vi "correction_beamshaper_example.vi"() -> ()   [LabVIEW 2020, in "ILAO_BeamShaper.lvclass"]
uses:
  ILAO_BeamShaper/ILAO_BeamShaper.lvclass
  HASO4_3/WaveKit/Controls/InteractionMatrixToCommandMatrixParameters.ctl
  HASO4_3/WaveKit/Classes/CorrectionDataManager/CorrectionDataManager.lvclass
  HASO4_3/WaveKit/Classes/Pupil/Pupil.lvclass
  HASO4_3/WaveKit/Controls/Point2Df.ctl
  HASO4_3/WaveKit/Controls/CircularPupilDetectionParams.ctl
  HASO4_3/WaveKit/Controls/PupilDetectionOption.ctl
  HASO4_3/WaveKit/Controls/CircularAutoDetectionOptions.ctl
  HASO4_3/WaveKit/Controls/PupilDetectionMode.ctl
  HASO4_3/WaveKit/Controls/WavefrontModalReconstructionType.ctl
  HASO4_3/WaveKit/Classes/ModalCoef/ModalCoef.lvclass
  HASO4_3/WaveKit/Classes/ComputePhaseSet/ComputePhaseSet.lvclass
  HASO4_3/WaveKit/Controls/WavefrontReconstructionMode.ctl
  HASO4_3/WaveKit/Classes/HasoSlopes/HasoSlopes.lvclass
  HASO4_3/WaveKit/Classes/WavefrontCorrector/WavefrontCorrector.lvclass
  HASO4_3/WaveKit/Controls/ZernikeModalPrefs.ctl
  HASO4_3/WaveKit/Controls/ZernikeProjectionPupilSetup.ctl
panel:
  in  "Interaction matrix path 2":path
  in  "Haso config file path 2":path
  in  "PathToWavefrontCorrectorSetupFile 2":path
  out "Delta commands 2":sgl[](graph)
  in  "Prefs 2":T1={"Number of kept modes"=32, "Tilt filtering"=FALSE}
  in  "Zernike Value 2":dbl[](array[numeric])=[0.0, 0.0, 0.0, 0.0, 0.0, 0.0, 0.0, 0.0, 0.0]
  in  "Normalization 2":bool
  in  "set_init_state_from_config_file":bool
  in  "PathToWavefrontCorrectorSetupFile":path
  out "error out":errorcluster
  out "Delta commands":sgl[](graph)
  in  "Prefs":T1={"Number of kept modes"=32, "Tilt filtering"=FALSE}
  in  "Zernike Value":dbl[](array[numeric])=[0.0, 0.0, 0.0, 0.0, 0.0, 0.0, 0.0, 0.0, 0.0]
  in  "Normalization":bool
  in  "Interaction matrix path":path
  in  "Haso config file path":path
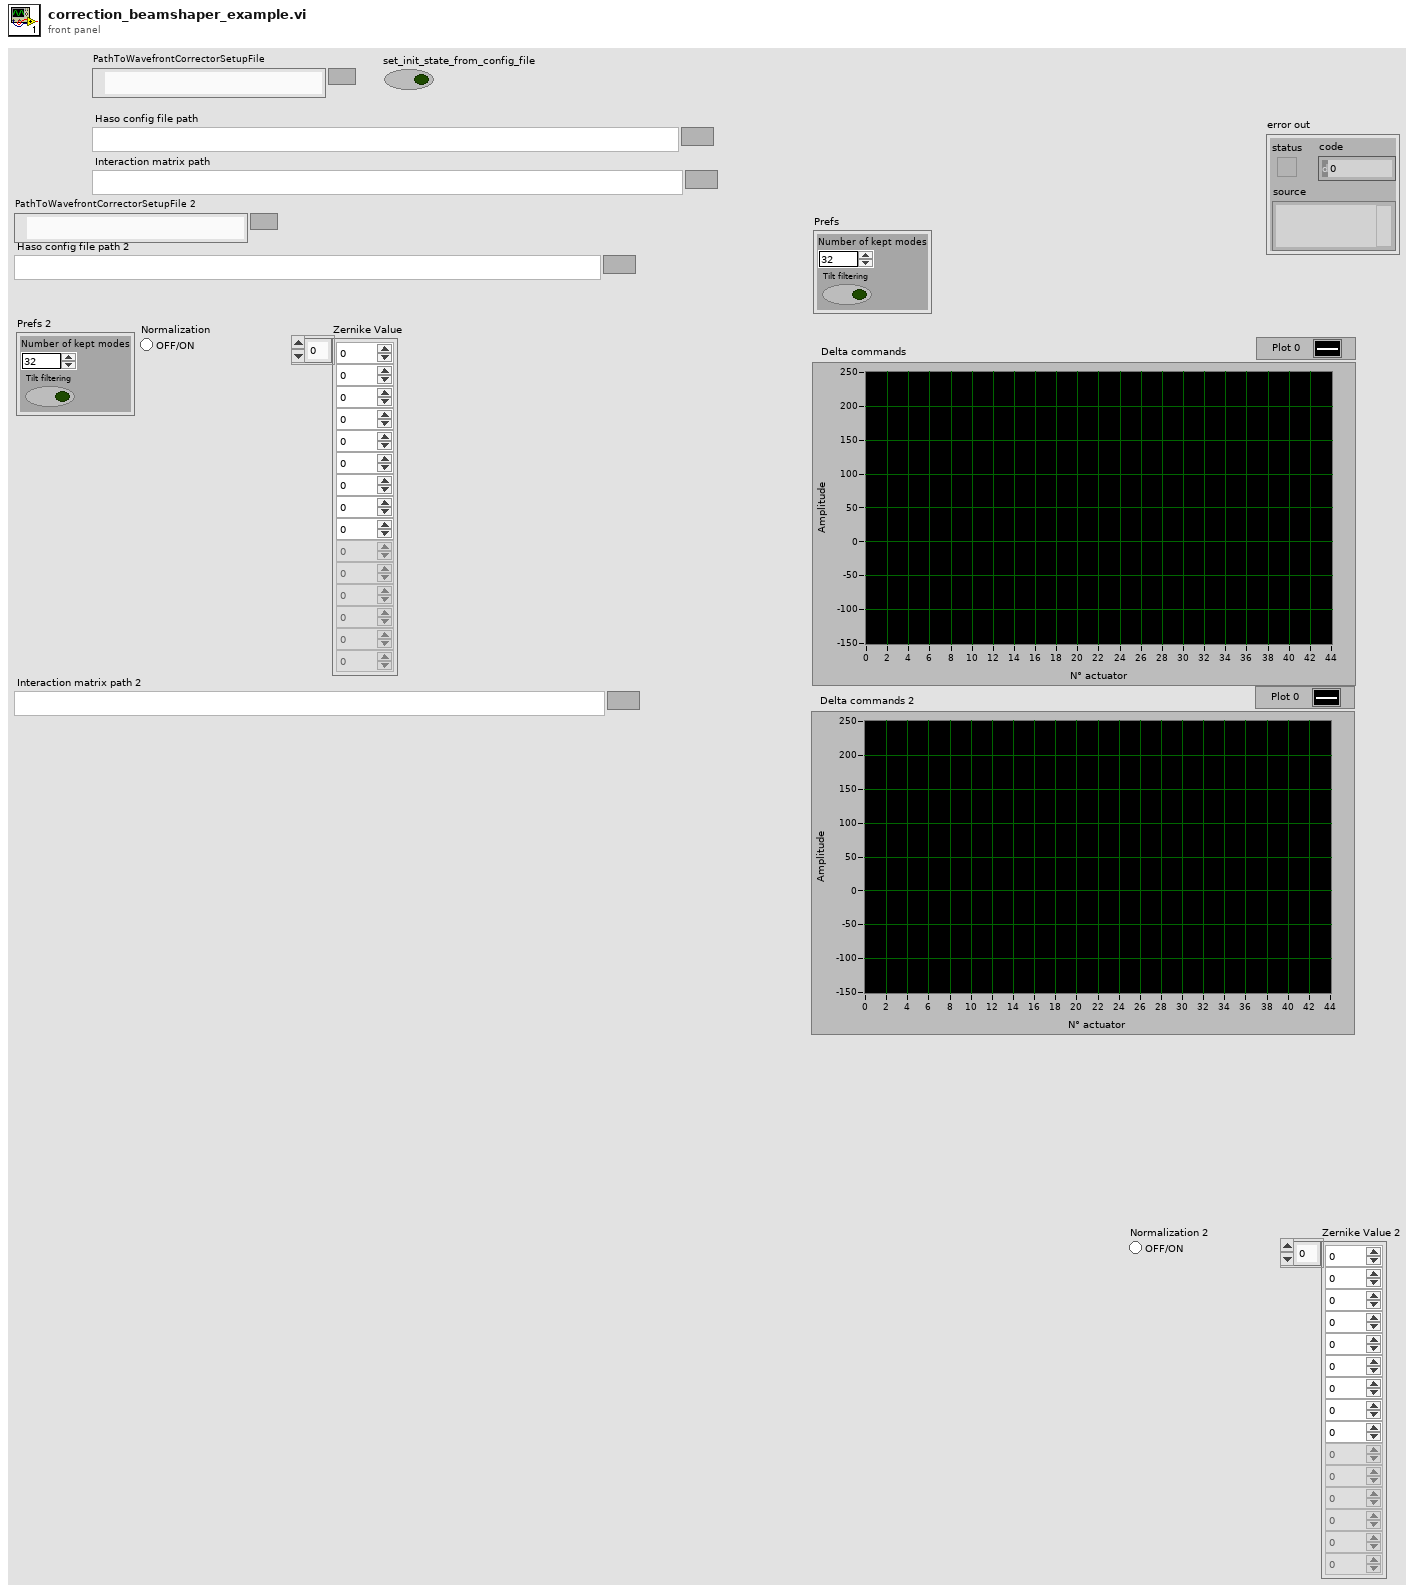
[diagram p1: front panel]
types:
  T1 = typedef "InteractionMatrixToCommandMatrixParameters.ctl" = cluster{"Number of kept modes":i32, "Tilt filtering":bool}
  T2 = typedef "ZernikeModalPrefs.ctl" = cluster{"Number of coefficients":u32, "Filtered coefficients":u32[], "RMS Zernike normalization":bool, "CircularProjectionPupilDimensions":T3}
  T3 = typedef "ZernikeProjectionPupilSetup.ctl" = cluster{"Pupil center_sspp":T4, "Pupil radius_sspp":sgl}
  T4 = typedef "Point2Df.ctl" = cluster{"X":sgl, "Y":sgl}
  T5 = typedef "WavefrontReconstructionMode.ctl" = enum16{"None", "Modal_Legendre", "Modal_Zernike", "Zonal", "Modal_Zonal_Zernike", "Modal_Zonal_Legendre"}
  T6 = typedef "WavefrontModalReconstructionType.ctl" = enum16{"Legendre", "Zernike"}
  T7 = typedef "CircularPupilDetectionParams.ctl" = cluster{"PupilDetectionOption":T8, "AutoDetectionOption":T9, "PupilDetectionMode":T10, "CentralOccultationDetection":bool}
  T8 = typedef "PupilDetectionOption.ctl" = enum16{"Manual", "Automatic"}
  T9 = typedef "CircularAutoDetectionOptions.ctl" = enum16{"manual_radius_auto_center", "manual_center_auto_radius", "auto_radius_auto_center"}
  T10 = typedef "PupilDetectionMode.ctl" = enum16{"inscribed", "circumscribed"}
  T11 = typedef "CasaoManagerGeneralSpecifications.ctl" = cluster{"Wavefront corrector name":string, "Wavefront corrector serial number":string, "Nb actuators":i32, "HASO serial number":string, "Dimension_um":T12}
  T12 = typedef "General dimensions definition.ctl" = cluster{"Size":T13, "Step":T4}
  T13 = typedef "Point2D.ctl" = cluster{"X":u32, "Y":u32}
  T14 = typedef "Wavefront Corrector Position.ctl" = sgl[]
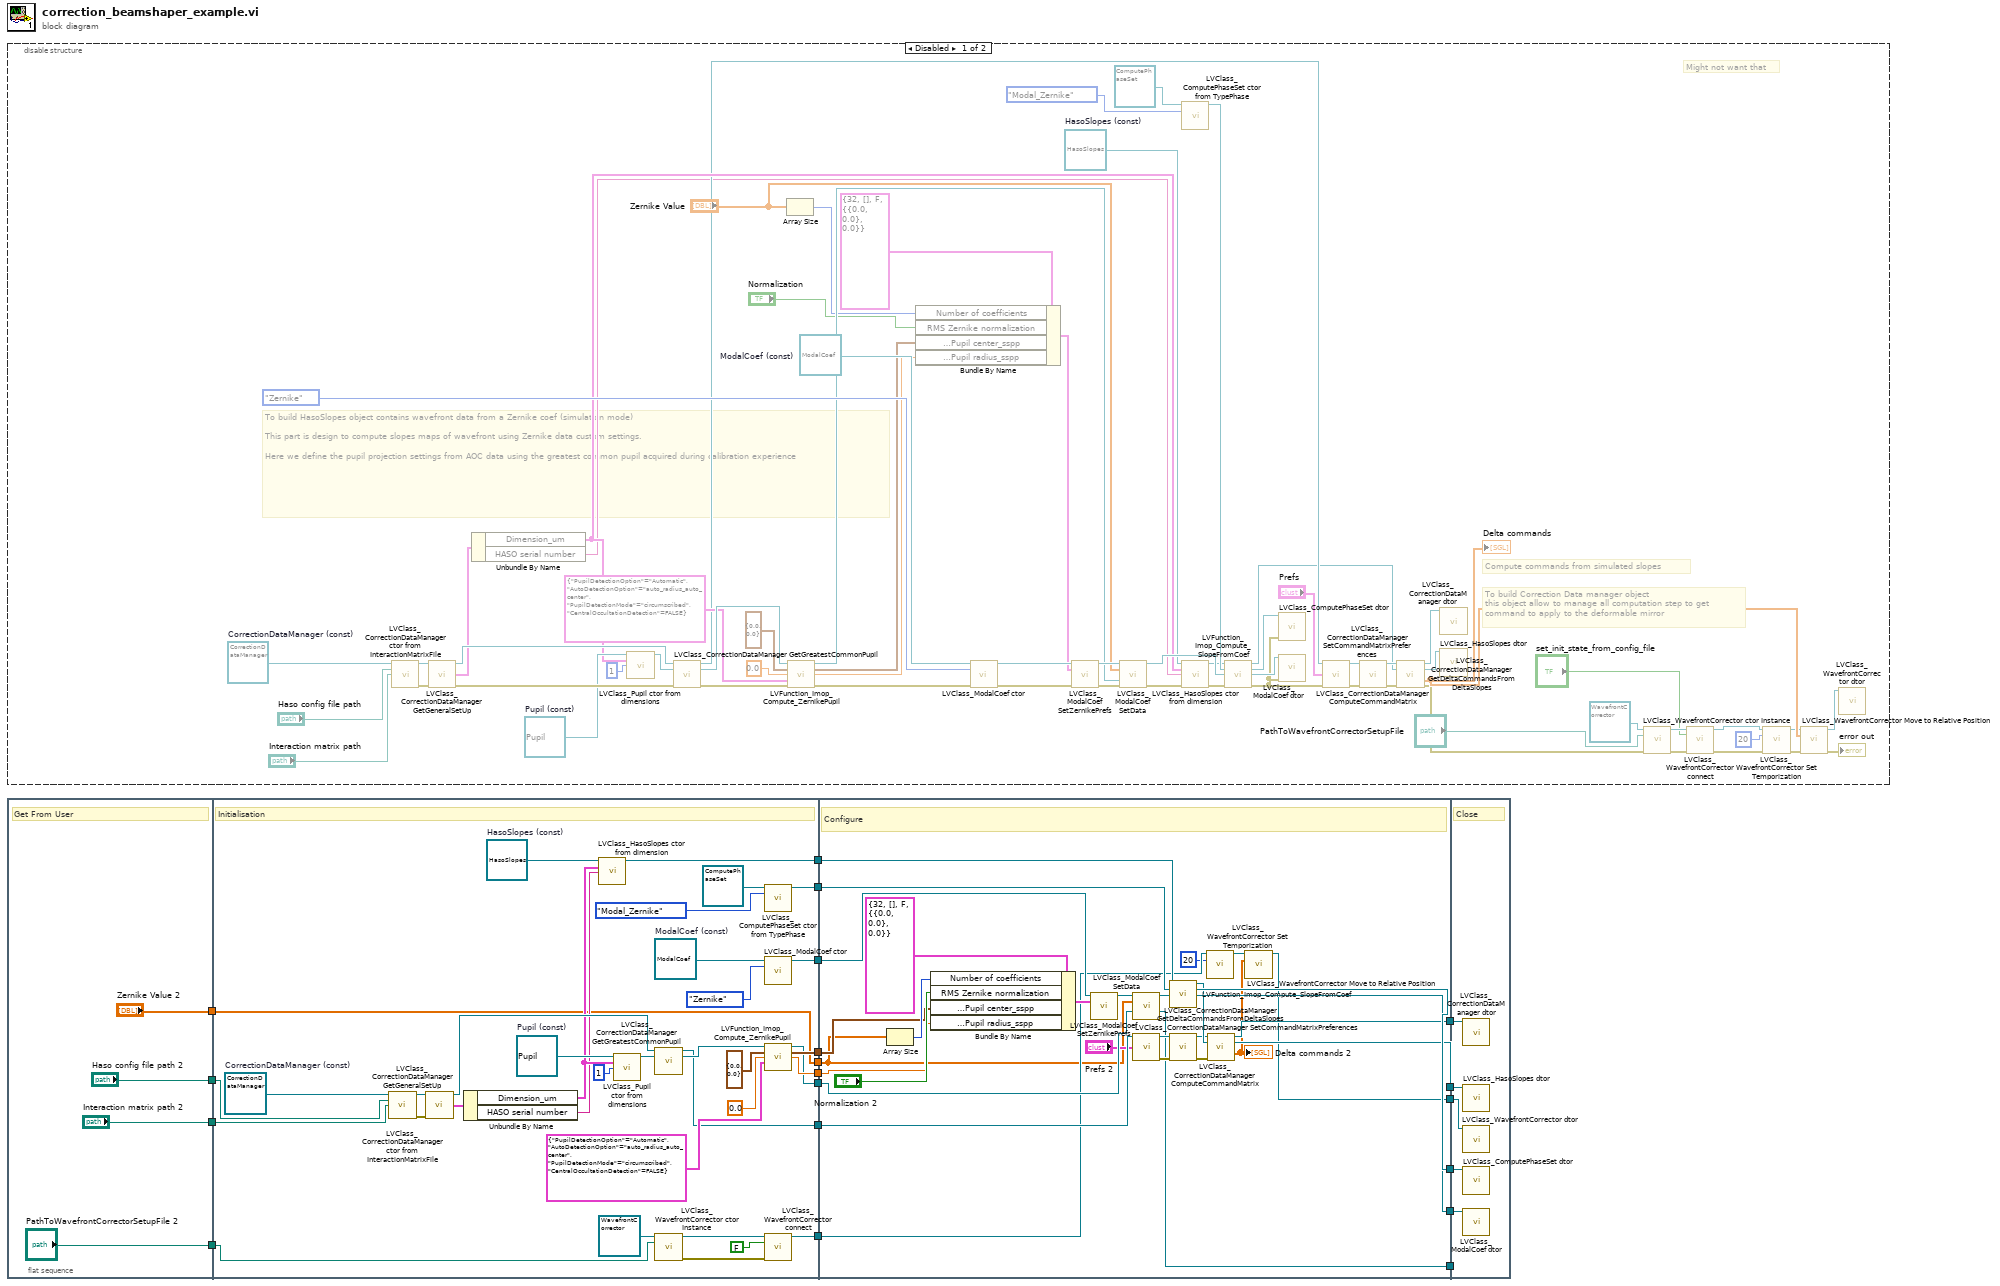
[diagram p0: block diagram]
diagram:
  n1 = disable-structure shown="Disabled" {
    frame Disabled {
      w49 = refnum<class "HasoSlopes.lvclass"> refnum  # HasoSlopes (const)
      w73 = refnum<class "ModalCoef.lvclass"> refnum  # ModalCoef (const)
      w80 = refnum<class "Pupil.lvclass"> refnum  # Pupil (const)
      w79 = refnum<class "CorrectionDataManager.lvclass"> refnum  # CorrectionDataManager (const)
      # "Might not want that"
      # "Compute commands from simulated slopes"
      # "To build HasoSlopes object contains wavefront data from a Zernike coef (simulation mode)\n\nThis part is design to compute slopes maps of wavefront using Zernike data custom settings.\n\nHere we define the pupil projection settings from AOC data using the greatest common pupil acquired during calibration experience"
      # "To build Correction Data manager object\nthis object allow to manage all computation step to get \ncommand to apply to the deformable mirror"
      n2 = call "LVClass_CorrectionDataManager ctor from InteractionMatrixFile.vi"("CorrectionDataManager (const)"=w79, "Haso config file path"="Haso config file path", "Interaction matrix path"="Interaction matrix path") -> ("CorrectionDataManager (new)"=w86:refnum<class "CorrectionDataManager.lvclass">, "error out"=w82:errorcluster)  [unwired: 11 in]
      n3 = call "LVClass_CorrectionDataManager GetGeneralSetUp.vi"("CorrectionDataManager in"=w86, "error in (no error)"=w82) -> ("CorrectionDataManager out"=w85:refnum<class "CorrectionDataManager.lvclass">, "general"=w60:T11, "error out"=w81:errorcluster)  [unwired: 11 in]
      n4 = Unbundle By Name(w60) -> ("Dimension_um"=w48:T12, "HASO serial number"=w36:string)
      n5 = call "LVClass_Pupil ctor from dimensions.vi"("Pupil (const)"=w80, "Dimensions_um"=w48, "value"=u8 1) -> ("Pupil (new)"=w83:refnum<class "Pupil.lvclass">)  [unwired: 11 in, 1 out]
      n6 = call "LVClass_CorrectionDataManager GetGreatestCommonPupil.vi"("CorrectionDataManager in"=w85, "Pupil in"=w83, "error in (no error)"=w81) -> ("CorrectionDataManager out"=w41:refnum<class "CorrectionDataManager.lvclass">, "Pupil out"=w76:refnum<class "Pupil.lvclass">, "error out"=w74:errorcluster)  [unwired: 10 in]
      n7 = Array Size(array="Zernike Value") -> (size(s)=w55:i32)
      n8 = call "LVFunction_Imop_Compute_ZernikePupil.vi"("Pupil.lvclass"=w76, "center in"=T4 {"X"=0.0, "Y"=0.0}, "radius in"=sgl 0.0, "CircularPupilDetectionParams"=T7 {"PupilDetectionOption"=enum."Automatic", "AutoDetectionOption"=enum."auto_radius_auto_center", "PupilDetectionMode"=enum."circumscribed", "CentralOccultationDetection"=FALSE}, "error in"=w74) -> ("Pupil.lvclass"=w58:refnum<class "Pupil.lvclass">, "center"=w51:T4, "radius"=w50:sgl, "error out"=w59:errorcluster)  [unwired: 7 in]
      n9 = Bundle By Name(cluster=T2 {"Number of coefficients"=32, "Filtered coefficients"=[], "RMS Zernike normalization"=FALSE, "CircularProjectionPupilDimensions"={"Pupil center_sspp"={"X"=0.0, "Y"=0.0}, "Pupil radius_sspp"=0.0}} ("ZernikeModalPrefs 2"), "Number of coefficients"=w55, "RMS Zernike normalization"="Normalization", "CircularProjectionPupilDimensions.Pupil center_sspp"=w51, "CircularProjectionPupilDimensions.Pupil radius_sspp"=w50) -> (w53:T2)
      n10 = call "LVClass_ModalCoef ctor.vi"("ModalCoef (const)"=w73, "TypePhase"=WavefrontModalReconstructionType."Zernike", "error in (no error)"=w59) -> ("ModalCoef (new)"=w71:refnum<class "ModalCoef.lvclass">, "error out"=w72:errorcluster)  [unwired: 11 in]
      n11 = call "LVClass_ModalCoef SetZernikePrefs.vi"("ModalCoef in"=w71, "ZernikeModalPrefs"=w53, "error in (no error)"=w72) -> ("ModalCoef out"=w70:refnum<class "ModalCoef.lvclass">, "error out"=w57:errorcluster)  [unwired: 11 in]
      n12 = call "LVClass_ModalCoef SetData.vi"("ModalCoef in"=w70, "coef"="Zernike Value", "Pupil.lvclass"=w58, "error in (no error)"=w57) -> ("ModalCoef out"=w64:refnum<class "ModalCoef.lvclass">, "error out"=w62:errorcluster)  [unwired: 8 in, 2 out]
      n13 = call "LVClass_ComputePhaseSet ctor from TypePhase.vi"("ComputePhaseSet (const)"=refnum<class "ComputePhaseSet.lvclass"> refnum ("ComputePhaseSet"), "TypePhase"=WavefrontReconstructionMode."Modal_Zernike") -> ("ComputePhaseSet (new)"=w63:refnum<class "ComputePhaseSet.lvclass">)  [unwired: 12 in, 1 out]
      n14 = call "LVClass_HasoSlopes ctor from dimension.vi"("HasoSlopes (const)"=w49, "Dimensions_um"=w48, "serial"=w36, "error in (no error)"=w62) -> ("HasoSlopes (new)"=w61:refnum<class "HasoSlopes.lvclass">, "error out"=w47:errorcluster)  [unwired: 10 in]
      n15 = call "LVFunction_Imop_Compute_SlopeFromCoef.vi"("HasoSlopes.lvclass"=w61, "ComputePhaseSet"=w63, "ModalCoef.lvclass"=w64, "error IO"=w47) -> ("HasoSlopes.lvclass"=w40:refnum<class "HasoSlopes.lvclass">, "ComputePhaseSet (dup)"=w65:refnum<class "ComputePhaseSet.lvclass">, "ModalCoef.lvclass (dup)"=w66:refnum<class "ModalCoef.lvclass">, "error IO out"=w39:errorcluster)  [unwired: 8 in]
      n16 = call "LVClass_ComputePhaseSet dtor.vi"("ComputePhaseSet in"=w65, "error in (no error)"=w39) -> ()  [unwired: 12 in, 2 out]
      n17 = call "LVClass_ModalCoef dtor.vi"("ModalCoef in"=w66, "error in (no error)"=w39) -> ()  [unwired: 12 in, 2 out]
      n18 = call "LVClass_CorrectionDataManager SetCommandMatrixPreferences.vi"("CorrectionDataManager in"=w41, "Prefs"="Prefs", "error in (no error)"=w39) -> ("CorrectionDataManager out"=w45:refnum<class "CorrectionDataManager.lvclass">, "error out"=w46:errorcluster)  [unwired: 11 in]
      n19 = call "LVClass_CorrectionDataManager ComputeCommandMatrix.vi"("CorrectionDataManager in"=w45, "error in (no error)"=w46) -> ("CorrectionDataManager out"=w44:refnum<class "CorrectionDataManager.lvclass">, "error out"=w43:errorcluster)  [unwired: 12 in]
      n20 = call "LVClass_CorrectionDataManager GetDeltaCommandsFromDeltaSlopes.vi"("CorrectionDataManager in"=w44, "Delta Slopes IN"=w40, "error in (no error)"=w43) -> ("CorrectionDataManager out"=w37:refnum<class "CorrectionDataManager.lvclass">, "Delta Slope OUT"=w38:refnum<class "HasoSlopes.lvclass">, "DeltaPosition"=w35:T14, "error out"=w25:errorcluster)  [unwired: 9 in]
      "Delta commands" <- w35
      n21 = call "LVClass_CorrectionDataManager dtor.vi"("CorrectionDataManager in"=w37) -> ()  [unwired: 13 in, 2 out]
      n22 = call "LVClass_HasoSlopes dtor.vi"("HasoSlopes in"=w38) -> ()  [unwired: 13 in, 2 out]
      n23 = call "LVClass_WavefrontCorrector ctor Instance.vi"("WavefrontCorrector (const)"=refnum<class "WavefrontCorrector.lvclass"> refnum ("WavefrontCorrector in"), "PathToWavefrontCorrectorSetupFile"="PathToWavefrontCorrectorSetupFile", "error in (no error)"=w25) -> ("WavefrontCorrector (new)"=w31:refnum<class "WavefrontCorrector.lvclass">, "error out"=w32:errorcluster)  [unwired: 11 in]
      n24 = call "LVClass_WavefrontCorrector connect.vi"("WavefrontCorrector in"=w31, "set_init_state_from_config_file"="set_init_state_from_config_file", "error in (no error)"=w32) -> ("WavefrontCorrector out"=w27:refnum<class "WavefrontCorrector.lvclass">, "error out"=w28:errorcluster)  [unwired: 11 in]
      n25 = call "LVClass_WavefrontCorrector Set Temporization.vi"("WavefrontCorrector in"=w27, "Sleep after command apply (ms)"=20, "error in (no error)"=w28) -> ("WavefrontCorrector out"=w22:refnum<class "WavefrontCorrector.lvclass">, "error out"=w24:errorcluster)  [unwired: 11 in]
      n26 = call "LVClass_WavefrontCorrector Move to Relative Position.vi"("WavefrontCorrector in"=w22, "Wavefront Relative Position"=w35, "error in (no error)"=w24) -> ("WavefrontCorrector out"=w33:refnum<class "WavefrontCorrector.lvclass">, "error out"=→"error out":errorcluster)  [unwired: 11 in]
      n27 = call "LVClass_WavefrontCorrector dtor.vi"("WavefrontCorrector in"=w33) -> ()  [unwired: 13 in, 2 out]
    }
    frame Enabled {
    }
  }
  n28 = flat-sequence {
    tunnel: ["Interaction matrix path 2"] -> w19
    tunnel: ["Haso config file path 2"] -> w18
    tunnel: ["PathToWavefrontCorrectorSetupFile 2"] -> w6
    tunnel: ["Zernike Value 2"] -> w2
    tunnel: w19 -> [w121]
    tunnel: w18 -> [w120]
    tunnel: [w111] -> w17
    tunnel: [w110] -> w16
    tunnel: [w107] -> w15
    tunnel: [w106] -> w14
    tunnel: [w100] -> w13
    tunnel: [w99] -> w12
    tunnel: [w98] -> w9
    tunnel: w6 -> [w96]
    tunnel: [w94] -> w5
    tunnel: [w91] -> w3
    tunnel: w2 -> [w91]
    tunnel: w17 -> [w152]
    tunnel: w16 -> [w151]
    tunnel: w15 -> [w150]
    tunnel: w14 -> [w147]
    tunnel: w13 -> [w145]
    tunnel: w12 -> [w146]
    tunnel: [w143] -> w11
    tunnel: [w142] -> w10
    tunnel: w9 -> [w139]
    tunnel: [w134] -> w8
    tunnel: [w133] -> w7
    tunnel: w5 -> [w131]
    tunnel: [w129] -> w4
    tunnel: w3 -> [w127]
    tunnel: [w126] -> w1
    tunnel: w11 -> [w160]
    tunnel: w10 -> [w159]
    tunnel: w8 -> [w158]
    tunnel: w7 -> [w157]
    tunnel: w4 -> [w156]
    tunnel: w1 -> [_]
    frame #0 {
      # "Get From User"
    }
    frame #1 {
      w103 = refnum<class "HasoSlopes.lvclass"> refnum  # HasoSlopes (const)
      w108 = refnum<class "ModalCoef.lvclass"> refnum  # ModalCoef (const)
      w118 = refnum<class "Pupil.lvclass"> refnum  # Pupil (const)
      w123 = refnum<class "CorrectionDataManager.lvclass"> refnum  # CorrectionDataManager (const)
      # "Initialisation"
      n29 = call "LVClass_CorrectionDataManager ctor from InteractionMatrixFile.vi"("CorrectionDataManager (const)"=w123, "Haso config file path"=w120, "Interaction matrix path"=w121) -> ("CorrectionDataManager (new)"=w125:refnum<class "CorrectionDataManager.lvclass">, "error out"=w124:errorcluster)  [unwired: 11 in]
      n30 = call "LVClass_CorrectionDataManager GetGeneralSetUp.vi"("CorrectionDataManager in"=w125, "error in (no error)"=w124) -> ("CorrectionDataManager out"=w119:refnum<class "CorrectionDataManager.lvclass">, "general"=w122:T11)  [unwired: 11 in, 1 out]
      n31 = Unbundle By Name(w122) -> ("Dimension_um"=w102:T12, "HASO serial number"=w101:string)
      n32 = call "LVClass_HasoSlopes ctor from dimension.vi"("HasoSlopes (const)"=w103, "Dimensions_um"=w102, "serial"=w101) -> ("HasoSlopes (new)"=w99:refnum<class "HasoSlopes.lvclass">)  [unwired: 11 in, 1 out]
      n33 = call "LVClass_Pupil ctor from dimensions.vi"("Pupil (const)"=w118, "Dimensions_um"=w102, "value"=u8 1) -> ("Pupil (new)"=w116:refnum<class "Pupil.lvclass">)  [unwired: 11 in, 1 out]
      n34 = call "LVClass_CorrectionDataManager GetGreatestCommonPupil.vi"("CorrectionDataManager in"=w119, "Pupil in"=w116) -> ("CorrectionDataManager out"=w98:refnum<class "CorrectionDataManager.lvclass">, "Pupil out"=w112:refnum<class "Pupil.lvclass">)  [unwired: 11 in, 1 out]
      n35 = call "LVClass_WavefrontCorrector ctor Instance.vi"("WavefrontCorrector (const)"=refnum<class "WavefrontCorrector.lvclass"> refnum ("WavefrontCorrector in"), "PathToWavefrontCorrectorSetupFile"=w96) -> ("WavefrontCorrector (new)"=w93:refnum<class "WavefrontCorrector.lvclass">, "error out"=w95:errorcluster)  [unwired: 12 in]
      n36 = call "LVClass_ComputePhaseSet ctor from TypePhase.vi"("ComputePhaseSet (const)"=refnum<class "ComputePhaseSet.lvclass"> refnum ("ComputePhaseSet"), "TypePhase"=WavefrontReconstructionMode."Modal_Zernike") -> ("ComputePhaseSet (new)"=w100:refnum<class "ComputePhaseSet.lvclass">)  [unwired: 12 in, 1 out]
      n37 = call "LVClass_ModalCoef ctor.vi"("ModalCoef (const)"=w108, "TypePhase"=WavefrontModalReconstructionType."Zernike") -> ("ModalCoef (new)"=w107:refnum<class "ModalCoef.lvclass">)  [unwired: 12 in, 1 out]
      n38 = call "LVFunction_Imop_Compute_ZernikePupil.vi"("Pupil.lvclass"=w112, "center in"=T4 {"X"=0.0, "Y"=0.0}, "radius in"=sgl 0.0, "CircularPupilDetectionParams"=T7 {"PupilDetectionOption"=enum."Automatic", "AutoDetectionOption"=enum."auto_radius_auto_center", "PupilDetectionMode"=enum."circumscribed", "CentralOccultationDetection"=FALSE}) -> ("Pupil.lvclass"=w106:refnum<class "Pupil.lvclass">, "center"=w111:T4, "radius"=w110:sgl)  [unwired: 8 in, 1 out]
      n39 = call "LVClass_WavefrontCorrector connect.vi"("WavefrontCorrector in"=w93, "set_init_state_from_config_file"=FALSE, "error in (no error)"=w95) -> ("WavefrontCorrector out"=w94:refnum<class "WavefrontCorrector.lvclass">)  [unwired: 11 in, 1 out]
    }
    frame #2 {
      # "Configure"
      n40 = Array Size(array=w127) -> (size(s)=w154:i32)
      n41 = Bundle By Name(cluster=T2 {"Number of coefficients"=32, "Filtered coefficients"=[], "RMS Zernike normalization"=FALSE, "CircularProjectionPupilDimensions"={"Pupil center_sspp"={"X"=0.0, "Y"=0.0}, "Pupil radius_sspp"=0.0}} ("ZernikeModalPrefs 2"), "Number of coefficients"=w154, "RMS Zernike normalization"="Normalization 2", "CircularProjectionPupilDimensions.Pupil center_sspp"=w152, "CircularProjectionPupilDimensions.Pupil radius_sspp"=w151) -> (w149:T2)
      n42 = call "LVClass_ModalCoef SetZernikePrefs.vi"("ModalCoef in"=w150, "ZernikeModalPrefs"=w149) -> ("ModalCoef out"=w148:refnum<class "ModalCoef.lvclass">)  [unwired: 12 in, 1 out]
      n43 = call "LVClass_ModalCoef SetData.vi"("ModalCoef in"=w148, "coef"=w127, "Pupil.lvclass"=w147) -> ("ModalCoef out"=w144:refnum<class "ModalCoef.lvclass">, "Pupil (dup)"=w126:refnum<class "Pupil.lvclass">)  [unwired: 9 in, 2 out]
      n44 = call "LVClass_CorrectionDataManager SetCommandMatrixPreferences.vi"("CorrectionDataManager in"=w139, "Prefs"="Prefs 2") -> ("CorrectionDataManager out"=w136:refnum<class "CorrectionDataManager.lvclass">, "error out"=w140:errorcluster)  [unwired: 12 in]
      n45 = call "LVFunction_Imop_Compute_SlopeFromCoef.vi"("HasoSlopes.lvclass"=w146, "ComputePhaseSet"=w145, "ModalCoef.lvclass"=w144) -> ("HasoSlopes.lvclass"=w137:refnum<class "HasoSlopes.lvclass">, "ComputePhaseSet (dup)"=w143:refnum<class "ComputePhaseSet.lvclass">, "ModalCoef.lvclass (dup)"=w142:refnum<class "ModalCoef.lvclass">)  [unwired: 9 in, 1 out]
      n46 = call "LVClass_CorrectionDataManager ComputeCommandMatrix.vi"("CorrectionDataManager in"=w136, "error in (no error)"=w140) -> ("CorrectionDataManager out"=w135:refnum<class "CorrectionDataManager.lvclass">, "error out"=w141:errorcluster)  [unwired: 12 in]
      n47 = call "LVClass_WavefrontCorrector Set Temporization.vi"("WavefrontCorrector in"=w131, "Sleep after command apply (ms)"=20) -> ("WavefrontCorrector out"=w132:refnum<class "WavefrontCorrector.lvclass">)  [unwired: 12 in, 1 out]
      n48 = call "LVClass_CorrectionDataManager GetDeltaCommandsFromDeltaSlopes.vi"("CorrectionDataManager in"=w135, "Delta Slopes IN"=w137, "error in (no error)"=w141) -> ("CorrectionDataManager out"=w133:refnum<class "CorrectionDataManager.lvclass">, "Delta Slope OUT"=w134:refnum<class "HasoSlopes.lvclass">, "DeltaPosition"=w130:T14)  [unwired: 9 in, 1 out]
      "Delta commands 2" <- w130
      n49 = call "LVClass_WavefrontCorrector Move to Relative Position.vi"("WavefrontCorrector in"=w132, "Wavefront Relative Position"=w130) -> ("WavefrontCorrector out"=w129:refnum<class "WavefrontCorrector.lvclass">)  [unwired: 12 in, 1 out]
    }
    frame #3 {
      # "Close"
      n50 = call "LVClass_CorrectionDataManager dtor.vi"("CorrectionDataManager in"=w157) -> ()  [unwired: 13 in, 2 out]
      n51 = call "LVClass_HasoSlopes dtor.vi"("HasoSlopes in"=w158) -> ()  [unwired: 13 in, 2 out]
      n52 = call "LVClass_WavefrontCorrector dtor.vi"("WavefrontCorrector in"=w156) -> ()  [unwired: 13 in, 2 out]
      n53 = call "LVClass_ComputePhaseSet dtor.vi"("ComputePhaseSet in"=w160) -> ()  [unwired: 13 in, 2 out]
      n54 = call "LVClass_ModalCoef dtor.vi"("ModalCoef in"=w159) -> ()  [unwired: 13 in, 2 out]
    }
  }
